vi "plot read scale refs.vi"(7 "Plot":refnum<vi>, 9 "RightAxisFocus":refnum<vi>, 11 "LeftAxisFocus":refnum<vi>) -> (0 "Right Scale":refnum<vi>, 1 "Left Scale":refnum<vi>, 2 "X Scale":refnum<vi>, 3 "Plot":refnum<vi>, 5 "Meta LUT":refnum<data-value>)   [LabVIEW 2021, in "RocketPlot.lvlib"]
uses:
  RocketPlot.lvlib
  TypeDefs/Plot axis.ctl
  TypeDefs/Plot scale meta JSON.ctl
  TypeDefs/Plot scale meta state.ctl
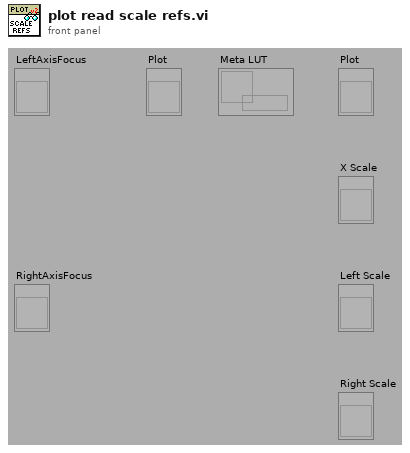
[diagram p1: front panel]
types:
  T1 = typedef "RocketPlot.lvlib/Plot axis.ctl" = enum16{"x axis", "left axis", "right axis"}
  T2 = typedef "RocketPlot.lvlib/Plot scale meta JSON.ctl" = cluster{"Type":T1, "Grid Colors:Major Color":u32, "Grid Colors:Minor Color":u32, "Style":u8, "Tick Colors:Tick Color":u32, "Tick Colors:Minor Tick Color":u32, "Format String":string, "State":T3, "AxisFocus":refnum<vi>}
  T3 = typedef "RocketPlot.lvlib/Plot scale meta state.ctl" = cluster{"Visible":bool, "Focus":bool, "Multi-Y":bool}
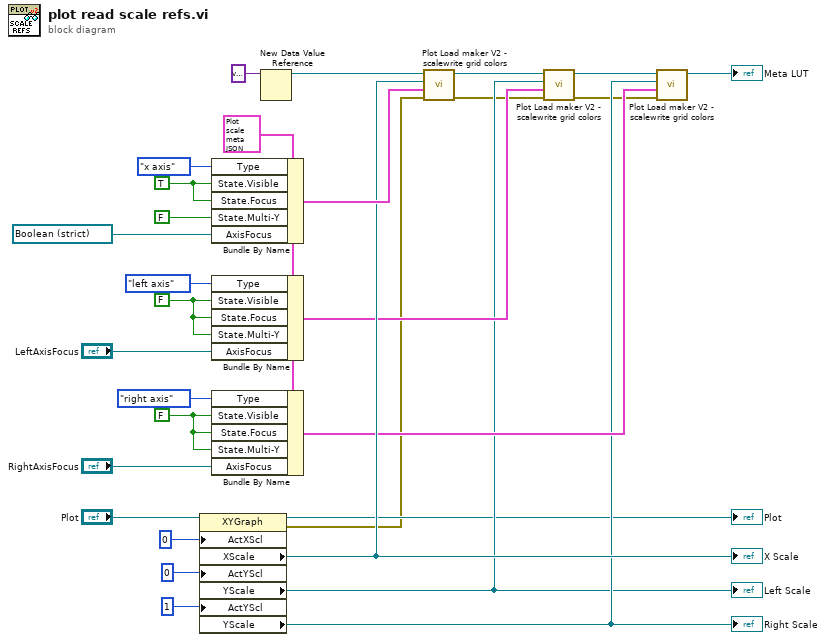
[diagram p0: block diagram]
diagram:
  w4 = FALSE ("State.Visible")
  w5 = FALSE ("State.Visible")
  w23 = TRUE ("State.Visible")
  w19 = T2 {"Type"=enum."x axis", "Grid Colors:Major Color"=0, "Grid Colors:Minor Color"=0, "Style"=0, "Tick Colors:Tick Color"=0, "Tick Colors:Minor Tick Color"=0, "Format String"="", "State"={"Visible"=FALSE, "Focus"=FALSE, "Multi-Y"=FALSE}, "AxisFocus"=refnum} ("Meta")
  n1 = property class="XYGraph"(reference="Plot", "ActXScl"=0 ("Active X Scale"), "ActYScl"=0 ("Active Y Scale"), "ActYScl"=1 ("Active Y Scale")) -> (reference out=→"Plot":refnum<vi>, error out=w9:errorcluster, "XScale"=w24:refnum<vi>, "YScale"=w11:refnum<vi>, "YScale"=w12:refnum<vi>)  [unwired: 1 in]
  "X Scale" <- w24
  "Left Scale" <- w11
  "Right Scale" <- w12
  n2 = Bundle By Name(cluster=w19, "Type"=Plot_axis."x axis", "State.Visible"=w23, "State.Focus"=w23, "State.Multi-Y"=FALSE, "AxisFocus"=refnum<vi> refnum) -> (w26:T2)
  n3 = Bundle By Name(cluster=w19, "Type"=Plot_axis."left axis", "State.Visible"=w5, "State.Focus"=w5, "State.Multi-Y"=w5, "AxisFocus"="LeftAxisFocus") -> (w16:T2)
  n4 = Bundle By Name(cluster=w19, "Type"=Plot_axis."right axis", "State.Visible"=w4, "State.Focus"=w4, "State.Multi-Y"=w4, "AxisFocus"="RightAxisFocus") -> (w15:T2)
  n5 = New Data Value Reference(data value=variant) -> (data value reference=w25:refnum<data-value>)  [unwired: 1 in, 1 out]
  n6 = call "Plot Load maker V2 - scalewrite grid colors.vi"("error in (no error)"=w9, "Meta"=w26, "Scale reference"=w24, "Meta LUT"=w25) -> ("error out"=w8:errorcluster, "Meta LUT"=w18:refnum<data-value>)  [unwired: 5 in, 1 out]
  n7 = call "Plot Load maker V2 - scalewrite grid colors.vi"("error in (no error)"=w8, "Meta"=w16, "Scale reference"=w11, "Meta LUT"=w18) -> ("error out"=w7:errorcluster, "Meta LUT"=w17:refnum<data-value>)  [unwired: 5 in, 1 out]
  n8 = call "Plot Load maker V2 - scalewrite grid colors.vi"("error in (no error)"=w7, "Meta"=w15, "Scale reference"=w12, "Meta LUT"=w17) -> ("Meta LUT"=→"Meta LUT":refnum<data-value>)  [unwired: 5 in, 2 out]
